vi "ReusePeakLocation.vi"(9 "MaxIndex in":i32, 10 "Tone In":T2={"Shift_"=0.0, "Peak_ToFPGA"=0.0, "MaxValue"=0.0, "MaxIndex"=0, "Tone"={"PkLocTrak"=0.0, "PkLocDisp"=0.0, "df_"=0.0, "ZoomPwr"=[], "Phase"=0.0, "PhaseOld"=0.0, "AboveThresh?"=FALSE, "MaxI"=0.0, "MaxQ"=0.0, "median"=0.0, "ISpect"=[], "QSpect"=[], "DeltaPhase"=0.0}, "TimeDomainI"=[], "TimeDomainQ"=[], "PwrSpectrum"=[], "RunningAvgFreq"=0.0, "ISpectPos"=[], "ISpectNeg"=[], "QSpectPos"=[], "QSpectNeg"=[], "10Hz_PwrSpectr"=[], "SNR"=0.0, "AliasWarn"=FALSE, "10Hz_Peak"=[], "ISpect+-"=[], "QSpect+-"=[], "TimeStamp"=timestamp(0 s since 1904-01-01), "I_Index"=array[12500 elements], "Q_Index"=array[12500 elements], "10MHz"=FALSE} {"Tone"."median" format="%0.2f"; "Tone"."MaxQ" format="%0.2f"}, 11 "Now.Target":T1) -> (3 "MaxIndex out":i32)   [LabVIEW 2018]
doc: "If this channel is one of the co-axis channels (channel 1 or channel 3) use the newly-found peak bin index location.\nIf this channel is one of the cross-axis channels (channel 2 or channel 4) use the previously-found peak bin index location.\nBecause the signal strength is greater with the co-axis channels, we want to use those channels to pick the peak location. The cross-axis bin locations are overwritten using co-axis values outside of this subVI."
uses:
  Controls/Clusts/ChannelToneData.ctl
  Controls/ToneInfoClust.ctl
  Controls/Enums/TargetNumber.ctl
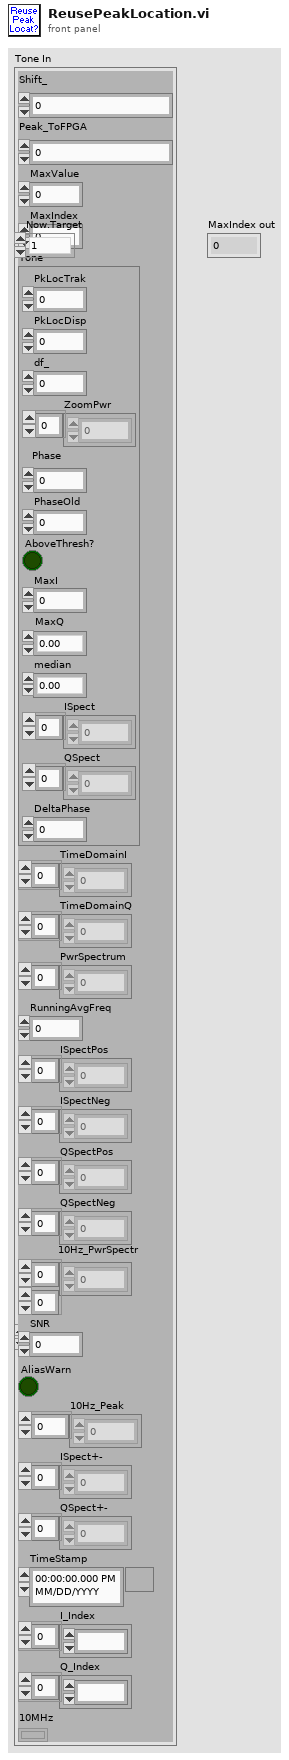
[diagram p1: front panel]
types:
  T1 = typedef "TargetNumber.ctl" = enum16{"1", "2", "3", "4"}
  T2 = typedef "ChannelToneData.ctl" = cluster{"Shift_":dbl, "Peak_ToFPGA":dbl, "MaxValue":dbl, "MaxIndex":i32, "Tone":T3, "TimeDomainI":ext[], "TimeDomainQ":ext[], "PwrSpectrum":dbl[], "RunningAvgFreq":dbl, "ISpectPos":dbl[], "ISpectNeg":dbl[], "QSpectPos":dbl[], "QSpectNeg":dbl[], "10Hz_PwrSpectr":dbl[][], "SNR":dbl, "AliasWarn":bool, "10Hz_Peak":dbl[], "ISpect+-":dbl[], "QSpect+-":dbl[], "TimeStamp":timestamp, "I_Index":ext[], "Q_Index":ext[], "10MHz":bool}
  T3 = typedef "ToneInfoClust.ctl" = cluster{"PkLocTrak":dbl, "PkLocDisp":dbl, "df_":dbl, "ZoomPwr":dbl[], "Phase":dbl, "PhaseOld":dbl, "AboveThresh?":bool, "MaxI":dbl, "MaxQ":dbl, "median":dbl, "ISpect":dbl[], "QSpect":dbl[], "DeltaPhase":dbl}
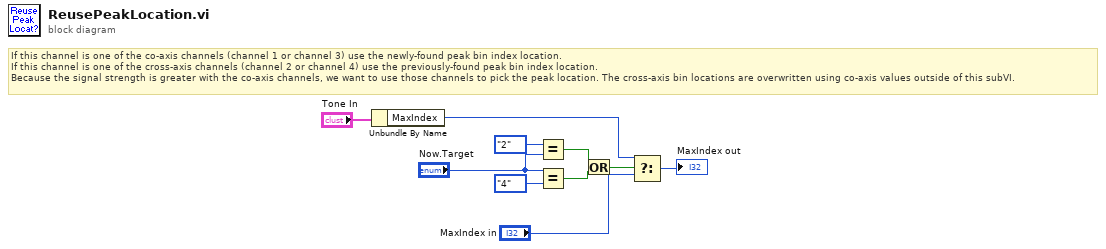
[diagram p0: block diagram]
diagram:
  # "If this channel is one of the co-axis channels (channel 1 or channel 3) use the newly-found peak bin index location.\nIf this channel is one of the cross-axis channels (channel 2 or channel 4) use the previously-found peak bin index location.\nBecause the signal strength is greater with the co-axis channels, we want to use those channels to pick the peak location. The cross-axis bin locations are overwritten using co-axis values outside of this subVI."
  n1 = Unbundle By Name("Tone In") -> ("MaxIndex"=w8:i32)
  n2 = Equal?(x=TargetNumber."2", y="Now.Target") -> (x = y?=w1:bool)
  n3 = Equal?(x="Now.Target", y=TargetNumber."4") -> (x = y?=w2:bool)
  n4 = Or(x=w1, y=w2) -> (x .or. y?=w7:bool)
  n5 = Select(t=w8, s=w7, f="MaxIndex in") -> (s? t:f=→"MaxIndex out":i32)
